vi "Run.vi"(7 "Team Index":i32, 8 "Column":i32, 9 "Row":i32, 10 "View":i32[](array[numeric]) caption="View (Team Index, -1: empty)", 11 "Swirl In":refnum<class "Swirl.lvclass">) -> (0 "Replicated":refnum<class "Square.lvclass">, 1 "Direction":T1, 2 "Action":T2, 3 "Swirl Out":refnum<class "Swirl.lvclass">)   [LabVIEW 2015, in "Swirl.lvclass"]
uses:
  Swirl.lvclass
  Type Defs/Action Enum.ctl
  Type Defs/Direction Enum.ctl
  Square/Square.lvclass
  SubVIs/Read-Only Globals.vi
  SubVIs/Globals (private).vi
  Common/Common.lvlib
  Type Defs/SB Type Defs.lvlib
panel:
  # "NW\nN\nNE\nE\nSE\nS\nSW\nW"
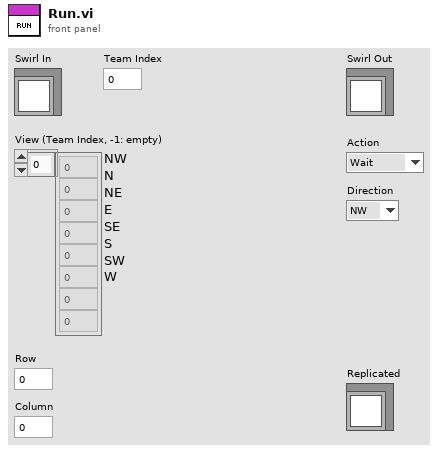
[diagram p1: front panel]
types:
  T1 = typedef "SB Type Defs.lvlib/Direction Enum.ctl" = enum16{"NW", "N", "NE", "E", "SE", "S", "SW", "W"}
  T2 = typedef "SB Type Defs.lvlib/Action Enum.ctl" = enum16{"Wait", "Move", "Attack", "Replicate"}
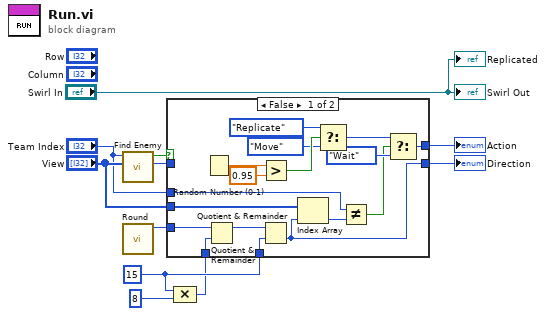
[diagram p0: block diagram]
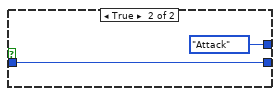
[diagram p2: hidden frame]
diagram:
  w3 = 15 ("y")
  n1 = call "Find Enemy.vi"("View"="View", "Team Index"="Team Index") -> ("Numeric"=w9:i32, "Boolean"=w10:bool)  [unwired: 8 in]
  n2 = call "Round.vi"() -> ("Round"=w6:i32)  [unwired: 11 in]
  n3 = Compound Arithmetic op=MULTIPLY(w3, 8 ("value")) -> (w2:i32)
  n4 = case shown="False" w10 {
    tunnel: [w21 Action_Enum."Attack" ("Action")] -> w8
    tunnel: w9 -> [_ w29]
    tunnel: [w14 w29] -> w7
    tunnel: w6 -> [w23 _]
    tunnel: "View" -> [w19 _]
    tunnel: "Team Index" -> [w16 _]
    tunnel: w3 -> [w13 _]
    tunnel: w2 -> [w12 _]
    frame False {
      n5 = Random Number (0-1)() -> (number: 0 to 1=w28:dbl)
      n6 = Quotient & Remainder(x=w23, y=w12) -> (x-y*floor(x/y)=w15:i32)  [unwired: 1 out]
      n7 = Greater?(x=w28, y=0.95) -> (0:w26:bool)
      n8 = Quotient & Remainder(x=w15, y=w13) -> (floor(x/y)=w14:i32)  [unwired: 1 out]
      n9 = Index Array(array=w19, index=w14) -> (element=w18:i32)
      n10 = Select(t=Action_Enum."Replicate" ("Action"), s=w26, f=Action_Enum."Move" ("Action")) -> (s? t:f=w22:T2)
      n11 = Not Equal?(x=w16, y=w18) -> (x != y?=w17:bool)
      n12 = Select(t=w22, s=w17, f=Action_Enum."Wait" ("Action")) -> (s? t:f=w21:T2)
    }
    frame True {
    }
  }
  "Action" <- w8
  "Direction" <- w7
  "Swirl Out" <- "Swirl In"
  "Replicated" <- "Swirl In"
